vi "Versioned Load.vi"(8 "Traj Info":T5 {"Cluster 2"."Limits"."StoopidFast (fps)" min=0.0; "Cluster 2"."Limits"."Jerk (fps^3)" min=0.0 step=1.0; "Cluster 2"."Limits"."Accel (fps^2)" min=0.0; "Cluster 2"."Limits"."Velocity (fps)" min=0.0}, 10 "path":path) -> (0 "Reversals":T6, 1 "Trajectory Data":T1(array[cluster]), 2 "Zero V":bool, 3 "Commands out":cluster{"Time (s)":dbl, T3, bool}[](array[cluster]), 4 "Fields":T7, 5 "Points out":cluster{"x":dbl, "y":dbl, "th":dbl}[](array[cluster]), 7 "Overall":cluster{"Time (s)":dbl, "Distance (ft)":dbl})   [LabVIEW 2019]
uses:
  Types/Single Cmd Info.ctl
  <vilib>/picture/picture.llb/imagedata.ctl
  Types/Limits.ctl
  Types/Availible Command systems for auto.ctl
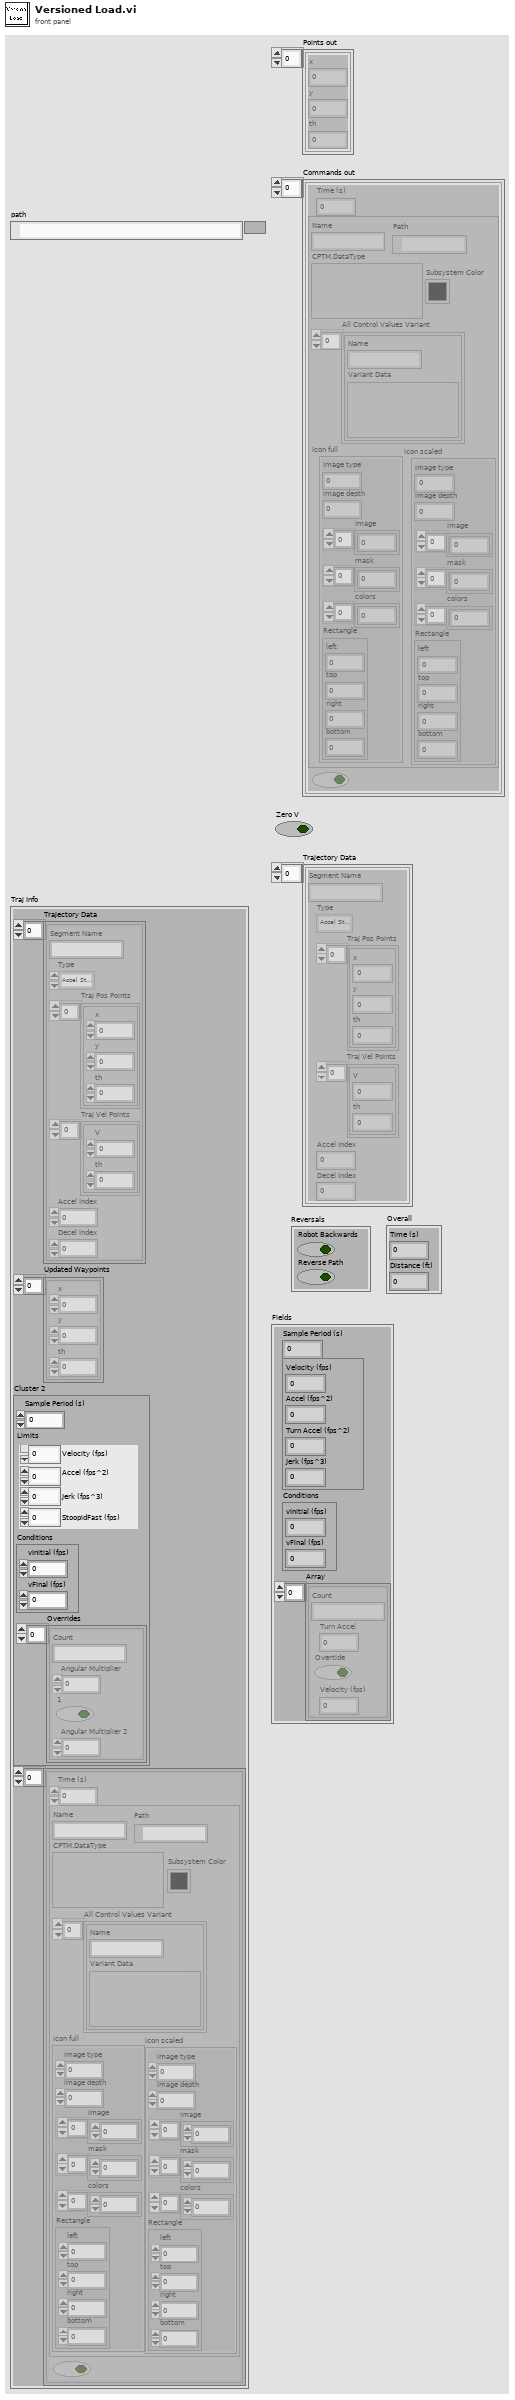
[diagram p1: front panel]
types:
  T1 = cluster{"Segment Name":string, "Type":enum16{"Accel Straight", "Const Straight", "Blend", "Circle"}, "Traj Pos Points":cluster{"x":dbl, "y":dbl, "th":dbl}[], "Traj Vel Points":cluster{"V":dbl, "th":dbl}[], "Accel Index":i32, "Decel Index":i32}[]
  T2 = typedef "Limits.ctl" = cluster{"Velocity (fps)":dbl, "Accel (fps^2)":dbl, "Jerk (fps^3)":dbl, "StoopidFast (fps)":dbl}
  T3 = typedef "Single Cmd Info.ctl" = cluster{"Name":string, "CPTM.DataType":variant, "All Control Values Variant":cluster{"Name":string, "Variant Data":variant}[], "icon full":T4, "icon scaled":T4, "Path":path, "Subsystem Color":u32}
  T4 = typedef "imagedata.ctl" = cluster{"image type":i32, "image depth":i32, "image":u8[], "mask":u8[], "colors":u32[], "Rectangle":cluster{"left":i16, "top":i16, "right":i16, "bottom":i16}}
  T5 = cluster{"Trajectory Data":cluster{"Segment Name":string, "Type":enum16{"Accel Straight", "Const Straight", "Blend", "Circle"}, "Traj Pos Points":cluster{"x":dbl, "y":dbl, "th":dbl}[], "Traj Vel Points":cluster{"V":dbl, "th":dbl}[], "Accel Index":i32, "Decel Index":i32}[], "Updated Waypoints":cluster{"x":dbl, "y":dbl, "th":dbl}[], "Cluster 2":cluster{"Sample Period (s)":dbl, "Limits":T2, "Conditions":cluster{"vInitial (fps)":dbl, "vFinal (fps)":dbl}, "Overrides":cluster{"Count":string, "Angular Multiplier":dbl, "1":bool, "Angular Multiplier 2":dbl}[]}, cluster{"Time (s)":dbl, T3, bool}[]}
  T6 = cluster{"Robot Backwards":bool, "Reverse Path":bool}
  T7 = cluster{"Sample Period (s)":dbl, cluster{"Velocity (fps)":dbl, "Accel (fps^2)":dbl, "Turn Accel (fps^2)":dbl, "Jerk (fps^3)":dbl}, "Conditions":cluster{"vInitial (fps)":dbl, "vFinal (fps)":dbl}, "Array":cluster{"Count":string, "Turn Accel":dbl, "Overtide":bool, "Velocity (fps)":dbl}[]}
  T8 = cluster{"Sample Period (s)":dbl, "Limits 2":cluster{"Velocity (fps)":dbl, "Acceleration (fps^2)":dbl, "Jerk (fps^3)":dbl}, "Conditions":cluster{"vInitial (fps)":dbl, "vFinal (fps)":dbl}, " Acceleration Overrides":cluster{"Angular \nAccelerations":dbl[], "Accel Override Bools":bool[]}}
  T9 = cluster{"Count":string, "Angular Multiplier":dbl, "1":bool, "Angular Multiplier 2":dbl}[]
  T10 = cluster{"Velocity":dbl, "Sample Time":dbl, "Accel":dbl}
  T11 = cluster{"Sample Period (s)":dbl, "Limits":cluster{"Velocity (fps)":dbl, "Acceleration (fps^2)":dbl, "Jerk (fps^3)":dbl}, "Conditions":cluster{"vInitial (fps)":dbl, "vFinal (fps)":dbl}}
  T12 = cluster{"Sample Period (s)":dbl, "Limits":cluster{"Velocity (fps)":dbl, "Acceleration (fps^2)":dbl, "Jerk (fps^3)":dbl}, "Conditions":cluster{"vInitial (fps)":dbl, "vFinal (fps)":dbl}, "Min Rads":dbl[]}
  T13 = typedef "Availible Command systems for auto.ctl" = u16
  T14 = cluster{"Time into Path":dbl, "System":T13, "Item Selected?":bool, "System Selection":T13}[]
  T15 = cluster{"Sample Period (s)":dbl, "Limits 2":cluster{"Velocity (fps)":dbl, "Acceleration (fps^2)":dbl, "Jerk (fps^3)":dbl, "Stoopid Fast":dbl}, "Conditions":cluster{"vInitial (fps)":dbl, "vFinal (fps)":dbl}, " Acceleration Overrides":cluster{"Angular \nAccelerations":dbl[], "Accel Override Bools":bool[]}}
  T16 = cluster{"Sample Period (s)":dbl, "Limits":cluster{"Velocity (fps)":dbl, "Accel (fps^2)":dbl, "Turn Accel (fps^2)":dbl, "Jerk (fps^3)":dbl}, "Conditions":cluster{"vInitial (fps)":dbl, "vFinal (fps)":dbl}, cluster{dbl[], bool[]}}
  T17 = cluster{"Reverse Path":bool, "Robot Backwards":bool}
  T18 = cluster{"Velocity":dbl, "Accel":dbl, "Accel":dbl, "Velocity":dbl}
  T19 = cluster{"Velocity (fps)":dbl, "Acceleration (fps^2)":dbl, "Jerk (fps^3)":dbl}
  T20 = cluster{"vInitial (fps)":dbl, "vFinal (fps)":dbl}
  T21 = cluster{"Velocity (fps)":dbl, "Acceleration (fps^2)":dbl, "Jerk (fps^3)":dbl, "Velocity (fps)":dbl}
  T22 = cluster{string, "Angular Multiplier":dbl, bool, "Velocity (fps)":dbl}
  T23 = cluster{"Angular \nAccelerations":dbl[], "Accel Override Bools":bool[]}
  T24 = cluster{string, "Turn Accel":dbl, "Overtide":bool, "Velocity (fps)":dbl}[]
  T25 = cluster{"Velocity (fps)":dbl, "Acceleration (fps^2)":dbl, "Jerk (fps^3)":dbl, "Stoopid Fast":dbl}
  T26 = cluster{"Velocity (fps)":dbl, "Accel (fps^2)":dbl, "Turn Accel (fps^2)":dbl, "Jerk (fps^3)":dbl}
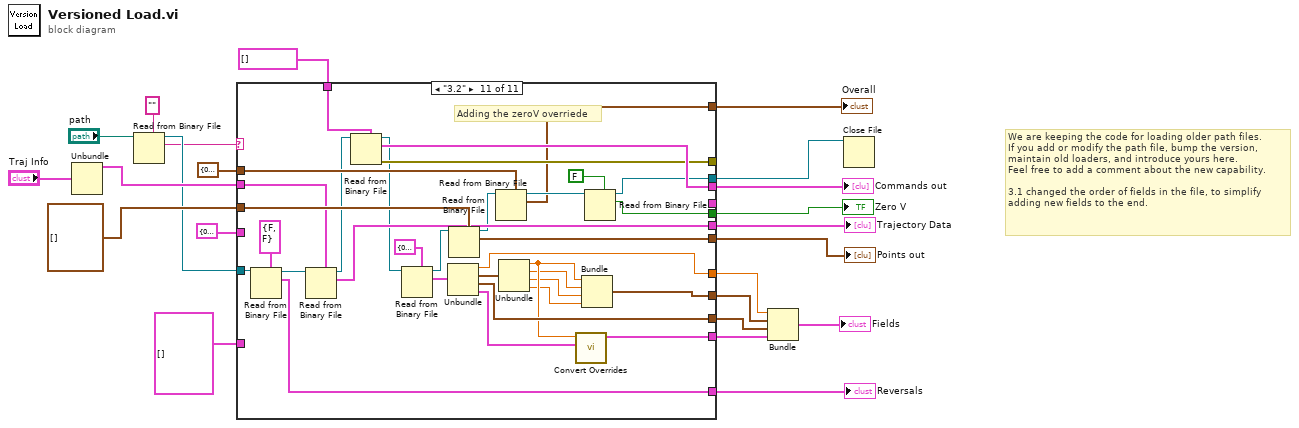
[diagram p0: block diagram]
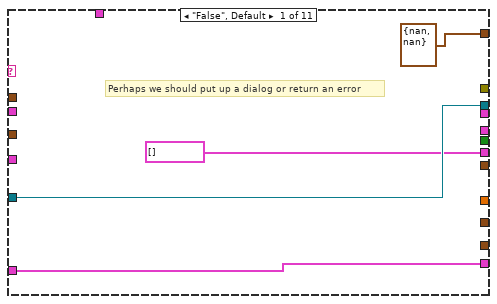
[diagram p2: hidden frame]
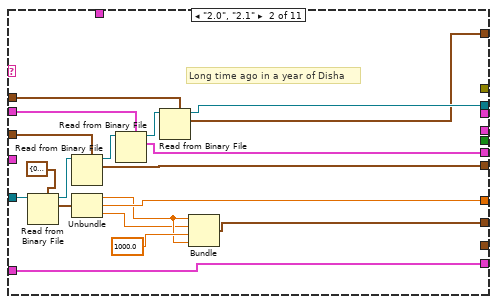
[diagram p3: hidden frame]
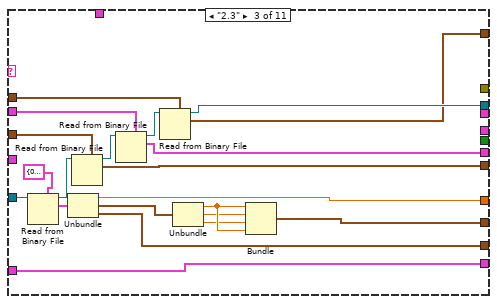
[diagram p4: hidden frame]
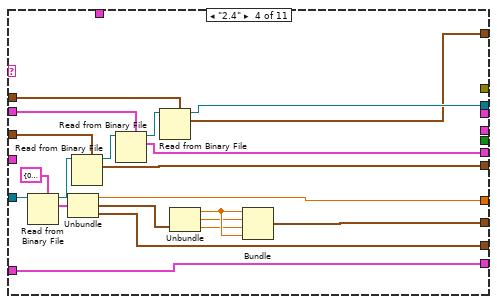
[diagram p5: hidden frame]
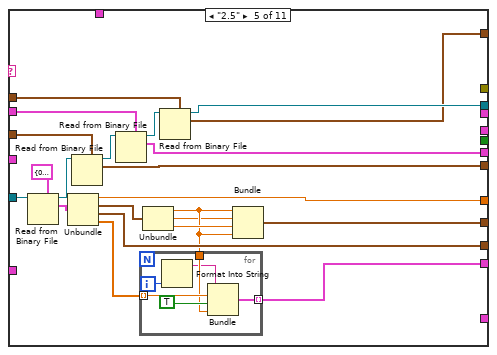
[diagram p6: hidden frame]
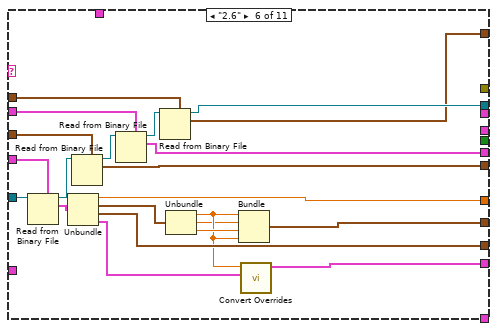
[diagram p7: hidden frame]
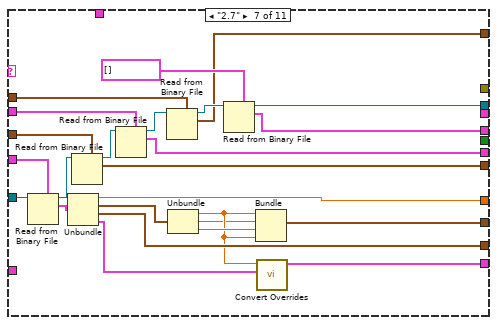
[diagram p8: hidden frame]
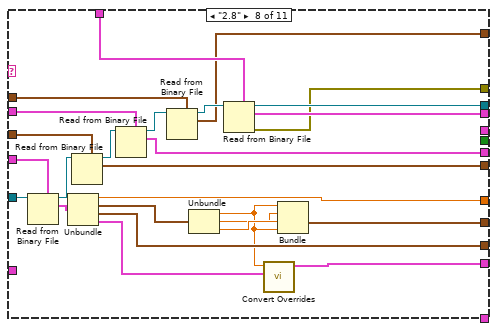
[diagram p9: hidden frame]
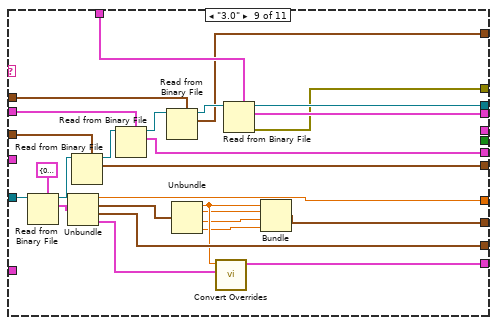
[diagram p10: hidden frame]
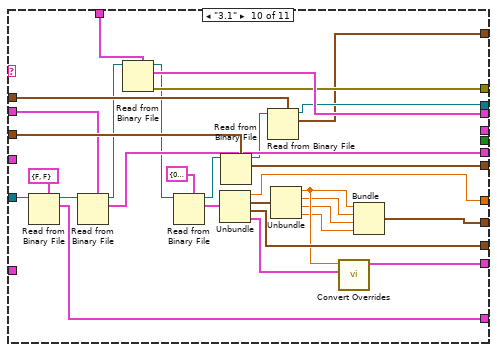
[diagram p11: hidden frame]
diagram:
  # "We are keeping the code for loading older path files.\nIf you add or modify the path file, bump the version,\nmaintain old loaders, and introduce yours here.\nFeel free to add a comment about the new capability.\n\n3.1 changed the order of fields in the file, to simplify\nadding new fields to the end."
  n1 = Unbundle("Traj Info") -> ("Trajectory Data"=w12:T1)  [unwired: 3 out]
  n2 = Read from Binary File(5:"" ("String"), 11:"path") -> (2:w3:string, 3:w4:refnum<file>)  [unwired: 4 in, 2 out]
  n3 = case shown="\"3.2\"" w3 {
    tunnel: w4 -> [w27 w45 w66 w87 w109 w137 w162 w188 w215 w235 w268]
    tunnel: cluster{"x":dbl, "y":dbl, "th":dbl}[] [] ("Points in") -> [_ w43 w64 w85 w107 w135 w160 w186 w213 w244 w277]
    tunnel: [_ w42 w63 w84 w106 w134 w159 w185 w212 w243 w276] -> w10
    tunnel: w12 -> [_ w41 w62 w83 w105 w133 w158 w184 w211 w242 w275]
    tunnel: cluster{"Time (s)":dbl, "Distance (ft)":dbl} {"Time (s)"=0.0, "Distance (ft)"=0.0} ("Cluster 4") -> [_ w39 w60 w81 w103 w131 w156 w182 w209 w241 w274]
    tunnel: [w27 w37 w58 w79 w101 w129 w150 w176 w203 w231 w250] -> w6
    tunnel: [_ w35 w57 w78 w100 w128 w154 w180 w207 w218 w252] -> w20
    tunnel: [_ w31 w51 w71 w94 w123 w144 w171 w191 w223 w257] -> w21
    tunnel: [_ _ w56 w77 w99 w127 w153 w179 w206 w240 w273] -> w22
    tunnel: [w25 w30 w50 w70 w93 w121 w141 w168 w197 w227 w261] -> w23
    tunnel: [T1 [] ("Trajectory Data") w33 w54 w75 w97 w126 w152 w178 w205 w239 w272] -> w9
    tunnel: [_ _ _ _ _ _ w149 _ _ _ _] -> _
    tunnel: cluster{"Time (s)":dbl, T3, bool}[] [] ("Commands in") -> [_ _ _ _ _ _ _ w175 w202 w238 w271]
    tunnel: [_ _ _ _ _ _ _ w174 w201 w237 w270] -> w14
    tunnel: [_ _ _ _ _ _ _ w173 w200 w236 w269] -> _
    tunnel: T8 {"Sample Period (s)"=0.0, "Limits 2"={"Velocity (fps)"=0.0, "Acceleration (fps^2)"=0.0, "Jerk (fps^3)"=0.0}, "Conditions"={"vInitial (fps)"=0.0, "vFinal (fps)"=0.0}, " Acceleration Overrides"={"Angular \nAccelerations"=[], "Accel Override Bools"=[]}} ("Cluster") -> [_ _ _ _ _ w125 w147 w169 _ _ _]
    tunnel: [_ _ _ _ _ _ _ _ _ w226 w260] -> w16
    tunnel: T9 [] ("Overrides") -> [w25 w30 w50 w70 _ _ _ _ _ _ _]
    tunnel: [_ _ _ _ _ _ _ _ _ _ w248] -> w18
    tunnel: [cluster{"Time (s)":dbl, "Distance (ft)":dbl} {"Time (s)"=nan, "Distance (ft)"=nan} ("Cluster 4") w28 w47 w68 w89 w117 w139 w164 w190 w217 w247] -> w1
    frame "False", Default {
      # "Perhaps we should put up a dialog or return an error"
    }
    frame "2.0", "2.1" {
      # "Long time ago in a year of Disha"
      n4 = Read from Binary File(5:T10 {"Velocity"=0.0, "Sample Time"=0.0, "Accel"=0.0}, 11:w45) -> (2:w46:T10, 3:w44:refnum<file>)  [unwired: 4 in, 2 out]
      n5 = Read from Binary File(5:w43, 11:w44) -> (2:w42:cluster{"x":dbl, "y":dbl, "th":dbl}[], 3:w40:refnum<file>)  [unwired: 4 in, 2 out]
      n6 = Unbundle(w46) -> ("Velocity"=w32:dbl, "Sample Time"=w35:dbl, "Accel"=w29:dbl)
      n7 = Read from Binary File(5:w41, 11:w40) -> (2:w33:T1, 3:w38:refnum<file>)  [unwired: 4 in, 2 out]
      n8 = Read from Binary File(5:w39, 11:w38) -> (2:w28:cluster{"Time (s)":dbl, "Distance (ft)":dbl}, 3:w37:refnum<file>)  [unwired: 4 in, 2 out]
      n9 = Bundle("Velocity"=w32, "Accel"=w29, "Accel"=1000.0, "Velocity"=w32) -> (w31:T18)  [unwired: 1 in]
    }
    frame "2.3" {
      n10 = Read from Binary File(5:T11 {"Sample Period (s)"=0.0, "Limits"={"Velocity (fps)"=0.0, "Acceleration (fps^2)"=0.0, "Jerk (fps^3)"=0.0}, "Conditions"={"vInitial (fps)"=0.0, "vFinal (fps)"=0.0}}, 11:w66) -> (2:w67:T11, 3:w65:refnum<file>)  [unwired: 4 in, 2 out]
      n11 = Unbundle(w67) -> ("Sample Period (s)"=w57:dbl, "Limits"=w48:T19, "Conditions"=w56:T20)
      n12 = Read from Binary File(5:w64, 11:w65) -> (2:w63:cluster{"x":dbl, "y":dbl, "th":dbl}[], 3:w61:refnum<file>)  [unwired: 4 in, 2 out]
      n13 = Read from Binary File(5:w62, 11:w61) -> (2:w54:T1, 3:w59:refnum<file>)  [unwired: 4 in, 2 out]
      n14 = Read from Binary File(5:w60, 11:w59) -> (2:w47:cluster{"Time (s)":dbl, "Distance (ft)":dbl}, 3:w58:refnum<file>)  [unwired: 4 in, 2 out]
      n15 = Unbundle(w48) -> ("Velocity (fps)"=w53:dbl, "Acceleration (fps^2)"=w49:dbl, "Jerk (fps^3)"=w52:dbl)
      n16 = Bundle("Velocity (fps)"=w53, "Acceleration (fps^2)"=w49, "Jerk (fps^3)"=w52, "Velocity (fps)"=w53) -> (w51:T21)  [unwired: 1 in]
    }
    frame "2.4" {
      n17 = Read from Binary File(5:T11 {"Sample Period (s)"=0.0, "Limits"={"Velocity (fps)"=0.0, "Acceleration (fps^2)"=0.0, "Jerk (fps^3)"=0.0}, "Conditions"={"vInitial (fps)"=0.0, "vFinal (fps)"=0.0}}, 11:w87) -> (2:w88:T11, 3:w86:refnum<file>)  [unwired: 4 in, 2 out]
      n18 = Unbundle(w88) -> ("Sample Period (s)"=w78:dbl, "Limits"=w72:T19, "Conditions"=w77:T20)
      n19 = Read from Binary File(5:w85, 11:w86) -> (2:w84:cluster{"x":dbl, "y":dbl, "th":dbl}[], 3:w82:refnum<file>)  [unwired: 4 in, 2 out]
      n20 = Read from Binary File(5:w83, 11:w82) -> (2:w75:T1, 3:w80:refnum<file>)  [unwired: 4 in, 2 out]
      n21 = Read from Binary File(5:w81, 11:w80) -> (2:w68:cluster{"Time (s)":dbl, "Distance (ft)":dbl}, 3:w79:refnum<file>)  [unwired: 4 in, 2 out]
      n22 = Unbundle(w72) -> ("Velocity (fps)"=w74:dbl, "Acceleration (fps^2)"=w69:dbl, "Jerk (fps^3)"=w73:dbl)
      n23 = Bundle("Velocity (fps)"=w74, "Acceleration (fps^2)"=w69, "Jerk (fps^3)"=w73, "Velocity (fps)"=w74) -> (w71:T21)  [unwired: 1 in]
    }
    frame "2.5" {
      n24 = Read from Binary File(5:T12 {"Sample Period (s)"=0.0, "Limits"={"Velocity (fps)"=0.0, "Acceleration (fps^2)"=0.0, "Jerk (fps^3)"=0.0}, "Conditions"={"vInitial (fps)"=0.0, "vFinal (fps)"=0.0}, "Min Rads"=[20.0, 20.0, 20.0, 20.0, 20.0]}, 11:w109) -> (2:w110:T12, 3:w108:refnum<file>)  [unwired: 4 in, 2 out]
      n25 = Unbundle(w110) -> ("Sample Period (s)"=w100:dbl, "Limits"=w95:T19, "Conditions"=w99:T20, "Min Rads"=w92:dbl[])
      n26 = Read from Binary File(5:w107, 11:w108) -> (2:w106:cluster{"x":dbl, "y":dbl, "th":dbl}[], 3:w104:refnum<file>)  [unwired: 4 in, 2 out]
      n27 = Read from Binary File(5:w105, 11:w104) -> (2:w97:T1, 3:w102:refnum<file>)  [unwired: 4 in, 2 out]
      n28 = Unbundle(w95) -> ("Velocity (fps)"=w91:dbl, "Acceleration (fps^2)"=w90:dbl, "Jerk (fps^3)"=w96:dbl)
      n29 = for {
        tunnel: [w115] -> w93 mode=indexing
        tunnel: w92 -> [w114] mode=indexing
        tunnel: w91 -> [w113]
        i -> [w112]
        n30 = Format Into String(w112) -> (resulting string=w111:string)  [unwired: 3 in, 1 out]
        n31 = Bundle(w111, "Angular Multiplier"=w114, TRUE, "Velocity (fps)"=w113) -> (w115:T22)  [unwired: 1 in]
      }
      n32 = Read from Binary File(5:w103, 11:w102) -> (2:w89:cluster{"Time (s)":dbl, "Distance (ft)":dbl}, 3:w101:refnum<file>)  [unwired: 4 in, 2 out]
      n33 = Bundle("Velocity (fps)"=w91, "Acceleration (fps^2)"=w90, "Jerk (fps^3)"=w96, "Velocity (fps)"=w91) -> (w94:T21)  [unwired: 1 in]
    }
    frame "2.6" {
      n34 = Read from Binary File(5:w125, 11:w137) -> (2:w138:T8, 3:w136:refnum<file>)  [unwired: 4 in, 2 out]
      n35 = Unbundle(w138) -> ("Sample Period (s)"=w128:dbl, "Limits 2"=w122:T19, "Conditions"=w127:T20, "Acceleration Overrides"=w119:T23)
      n36 = Read from Binary File(5:w135, 11:w136) -> (2:w134:cluster{"x":dbl, "y":dbl, "th":dbl}[], 3:w132:refnum<file>)  [unwired: 4 in, 2 out]
      n37 = Read from Binary File(5:w133, 11:w132) -> (2:w126:T1, 3:w130:refnum<file>)  [unwired: 4 in, 2 out]
      n38 = Read from Binary File(5:w131, 11:w130) -> (2:w117:cluster{"Time (s)":dbl, "Distance (ft)":dbl}, 3:w129:refnum<file>)  [unwired: 4 in, 2 out]
      n39 = Unbundle(w122) -> ("Velocity (fps)"=w120:dbl, "Acceleration (fps^2)"=w118:dbl, "Jerk (fps^3)"=w124:dbl)
      n40 = Bundle("Velocity (fps)"=w120, "Acceleration (fps^2)"=w118, "Jerk (fps^3)"=w124, "Velocity (fps)"=w120) -> (w123:T21)  [unwired: 1 in]
      n41 = call "Convert Overrides.vi"("Cluster"=w119, "Velocity (fps)"=w120) -> ("Array"=w121:T24)  [unwired: 9 in]
    }
    frame "2.7" {
      n42 = Read from Binary File(5:w147, 11:w162) -> (2:w163:T8, 3:w161:refnum<file>)  [unwired: 4 in, 2 out]
      n43 = Unbundle(w163) -> ("Sample Period (s)"=w154:dbl, "Limits 2"=w145:T19, "Conditions"=w153:T20, "Acceleration Overrides"=w142:T23)
      n44 = Read from Binary File(5:w160, 11:w161) -> (2:w159:cluster{"x":dbl, "y":dbl, "th":dbl}[], 3:w157:refnum<file>)  [unwired: 4 in, 2 out]
      n45 = Read from Binary File(5:w158, 11:w157) -> (2:w152:T1, 3:w155:refnum<file>)  [unwired: 4 in, 2 out]
      n46 = Read from Binary File(5:w156, 11:w155) -> (2:w139:cluster{"Time (s)":dbl, "Distance (ft)":dbl}, 3:w151:refnum<file>)  [unwired: 4 in, 2 out]
      n47 = Unbundle(w145) -> ("Velocity (fps)"=w143:dbl, "Acceleration (fps^2)"=w140:dbl, "Jerk (fps^3)"=w146:dbl)
      n48 = Read from Binary File(5:T14 [] ("Commands"), 11:w151) -> (2:w149:T14, 3:w150:refnum<file>)  [unwired: 4 in, 2 out]
      n49 = Bundle("Velocity (fps)"=w143, "Acceleration (fps^2)"=w140, "Jerk (fps^3)"=w146, "Velocity (fps)"=w143) -> (w144:T21)  [unwired: 1 in]
      n50 = call "Convert Overrides.vi"("Cluster"=w142, "Velocity (fps)"=w143) -> ("Array"=w141:T24)  [unwired: 9 in]
    }
    frame "2.8" {
      n51 = Read from Binary File(5:w169, 11:w188) -> (2:w189:T8, 3:w187:refnum<file>)  [unwired: 4 in, 2 out]
      n52 = Unbundle(w189) -> ("Sample Period (s)"=w180:dbl, "Limits 2"=w172:T19, "Conditions"=w179:T20, "Acceleration Overrides"=w166:T23)
      n53 = Read from Binary File(5:w186, 11:w187) -> (2:w185:cluster{"x":dbl, "y":dbl, "th":dbl}[], 3:w183:refnum<file>)  [unwired: 4 in, 2 out]
      n54 = Read from Binary File(5:w184, 11:w183) -> (2:w178:T1, 3:w181:refnum<file>)  [unwired: 4 in, 2 out]
      n55 = Read from Binary File(5:w182, 11:w181) -> (2:w164:cluster{"Time (s)":dbl, "Distance (ft)":dbl}, 3:w177:refnum<file>)  [unwired: 4 in, 2 out]
      n56 = Unbundle(w172) -> ("Velocity (fps)"=w167:dbl, "Acceleration (fps^2)"=w165:dbl, "Jerk (fps^3)"=w170:dbl)
      n57 = Read from Binary File(5:w175, 11:w177) -> (0:w173:errorcluster, 2:w174:cluster{"Time (s)":dbl, T3, bool}[], 3:w176:refnum<file>)  [unwired: 4 in, 1 out]
      n58 = call "Convert Overrides.vi"("Cluster"=w166, "Velocity (fps)"=w167) -> ("Array"=w168:T24)  [unwired: 9 in]
      n59 = Bundle("Velocity (fps)"=w167, "Acceleration (fps^2)"=w165, "Jerk (fps^3)"=w170, "Velocity (fps)"=w167) -> (w171:T21)  [unwired: 1 in]
    }
    frame "3.0" {
      n60 = Read from Binary File(5:T15 {"Sample Period (s)"=0.0, "Limits 2"={"Velocity (fps)"=0.0, "Acceleration (fps^2)"=0.0, "Jerk (fps^3)"=0.0, "Stoopid Fast"=0.0}, "Conditions"={"vInitial (fps)"=0.0, "vFinal (fps)"=0.0}, " Acceleration Overrides"={"Angular \nAccelerations"=[], "Accel Override Bools"=[]}} ("Cluster"), 11:w215) -> (2:w216:T15, 3:w214:refnum<file>)  [unwired: 4 in, 2 out]
      n61 = Unbundle(w216) -> ("Sample Period (s)"=w207:dbl, "Limits 2"=w192:T25, "Conditions"=w206:T20, "Acceleration Overrides"=w198:T23)
      n62 = Read from Binary File(5:w213, 11:w214) -> (2:w212:cluster{"x":dbl, "y":dbl, "th":dbl}[], 3:w210:refnum<file>)  [unwired: 4 in, 2 out]
      n63 = Read from Binary File(5:w211, 11:w210) -> (2:w205:T1, 3:w208:refnum<file>)  [unwired: 4 in, 2 out]
      n64 = Read from Binary File(5:w209, 11:w208) -> (2:w190:cluster{"Time (s)":dbl, "Distance (ft)":dbl}, 3:w204:refnum<file>)  [unwired: 4 in, 2 out]
      n65 = Unbundle(w192) -> ("Velocity (fps)"=w196:dbl, "Acceleration (fps^2)"=w195:dbl, "Jerk (fps^3)"=w194:dbl, "Stoopid Fast"=w193:dbl)
      n66 = call "Convert Overrides.vi"("Cluster"=w198, "Velocity (fps)"=w196) -> ("Array"=w197:T24)  [unwired: 9 in]
      n67 = Read from Binary File(5:w202, 11:w204) -> (0:w200:errorcluster, 2:w201:cluster{"Time (s)":dbl, T3, bool}[], 3:w203:refnum<file>)  [unwired: 4 in, 1 out]
      n68 = Bundle("Velocity (fps)"=w196, "Acceleration (fps^2)"=w195, "Jerk (fps^3)"=w194, "Stoopid Fast"=w193) -> (w191:T25)  [unwired: 1 in]
    }
    frame "3.1" {
      n69 = Read from Binary File(5:T17 {"Reverse Path"=FALSE, "Robot Backwards"=FALSE} ("Cluster"), 11:w235) -> (2:w226:T17, 3:w232:refnum<file>)  [unwired: 4 in, 2 out]
      n70 = Read from Binary File(5:w242, 11:w232) -> (2:w239:T1, 3:w230:refnum<file>)  [unwired: 4 in, 2 out]
      n71 = Read from Binary File(5:w238, 11:w230) -> (0:w236:errorcluster, 2:w237:cluster{"Time (s)":dbl, T3, bool}[], 3:w229:refnum<file>)  [unwired: 4 in, 1 out]
      n72 = Read from Binary File(5:T16 {"Sample Period (s)"=0.0, "Limits"={"Velocity (fps)"=0.0, "Accel (fps^2)"=0.0, "Turn Accel (fps^2)"=15.0, "Jerk (fps^3)"=0.0}, "Conditions"={"vInitial (fps)"=0.0, "vFinal (fps)"=0.0}, {[], []}} ("Cluster 2"), 11:w229) -> (2:w246:T16, 3:w245:refnum<file>)  [unwired: 4 in, 2 out]
      n73 = Unbundle(w246) -> ("Sample Period (s)"=w218:dbl, "Limits"=w225:T26, "Conditions"=w240:T20, w228:cluster{dbl[], bool[]})
      n74 = Read from Binary File(5:w244, 11:w245) -> (2:w243:cluster{"x":dbl, "y":dbl, "th":dbl}[], 3:w233:refnum<file>)  [unwired: 4 in, 2 out]
      n75 = Read from Binary File(5:w241, 11:w233) -> (2:w217:cluster{"Time (s)":dbl, "Distance (ft)":dbl}, 3:w231:refnum<file>)  [unwired: 4 in, 2 out]
      n76 = Unbundle(w225) -> ("Velocity (fps)"=w222:dbl, "Accel (fps^2)"=w221:dbl, "Turn Accel (fps^2)"=w220:dbl, "Jerk (fps^3)"=w219:dbl)
      n77 = call "Convert Overrides.vi"("Cluster"=w228, "Velocity (fps)"=w222) -> ("Array"=w227:T24)  [unwired: 9 in]
      n78 = Bundle("Velocity (fps)"=w222, "Accel (fps^2)"=w221, "Turn Accel (fps^2)"=w220, "Jerk (fps^3)"=w219) -> (w223:T26)  [unwired: 1 in]
    }
    frame "3.2" {
      # "Adding the zeroV overriede"
      n79 = Read from Binary File(5:T6 {"Robot Backwards"=FALSE, "Reverse Path"=FALSE} ("Cluster"), 11:w268) -> (2:w260:T6, 3:w265:refnum<file>)  [unwired: 4 in, 2 out]
      n80 = Read from Binary File(5:w275, 11:w265) -> (2:w272:T1, 3:w264:refnum<file>)  [unwired: 4 in, 2 out]
      n81 = Read from Binary File(5:w271, 11:w264) -> (0:w269:errorcluster, 2:w270:cluster{"Time (s)":dbl, T3, bool}[], 3:w263:refnum<file>)  [unwired: 4 in, 1 out]
      n82 = Read from Binary File(5:T16 {"Sample Period (s)"=0.0, "Limits"={"Velocity (fps)"=0.0, "Accel (fps^2)"=0.0, "Turn Accel (fps^2)"=15.0, "Jerk (fps^3)"=0.0}, "Conditions"={"vInitial (fps)"=0.0, "vFinal (fps)"=0.0}, {[], []}} ("Cluster 2"), 11:w263) -> (2:w279:T16, 3:w278:refnum<file>)  [unwired: 4 in, 2 out]
      n83 = Unbundle(w279) -> ("Sample Period (s)"=w252:dbl, "Limits"=w259:T26, "Conditions"=w273:T20, w262:cluster{dbl[], bool[]})
      n84 = Read from Binary File(5:w277, 11:w278) -> (2:w276:cluster{"x":dbl, "y":dbl, "th":dbl}[], 3:w266:refnum<file>)  [unwired: 4 in, 2 out]
      n85 = Read from Binary File(5:w274, 11:w266) -> (2:w247:cluster{"Time (s)":dbl, "Distance (ft)":dbl}, 3:w251:refnum<file>)  [unwired: 4 in, 2 out]
      n86 = Unbundle(w259) -> ("Velocity (fps)"=w256:dbl, "Accel (fps^2)"=w255:dbl, "Turn Accel (fps^2)"=w254:dbl, "Jerk (fps^3)"=w253:dbl)
      n87 = call "Convert Overrides.vi"("Cluster"=w262, "Velocity (fps)"=w256) -> ("Array"=w261:T24)  [unwired: 9 in]
      n88 = Bundle("Velocity (fps)"=w256, "Accel (fps^2)"=w255, "Turn Accel (fps^2)"=w254, "Jerk (fps^3)"=w253) -> (w257:T26)  [unwired: 1 in]
      n89 = Read from Binary File(5:FALSE, 11:w251) -> (2:w248:bool, 3:w250:refnum<file>)  [unwired: 4 in, 2 out]
    }
  }
  "Zero V" <- w18
  "Reversals" <- w16
  "Commands out" <- w14
  "Points out" <- w10
  "Trajectory Data" <- w9
  "Overall" <- w1
  n90 = Bundle("Sample Period (s)"=w20, w21, "Conditions"=w22, "Array"=w23) -> (→"Fields":T7)  [unwired: 1 in]
  n91 = Close File(refnum=w6) -> ()  [unwired: 1 in, 2 out]
